vi "Configure.vi"(8 "error in":errorcluster, 10 "name":string="CRDS", 11 "tCRD in":refnum<class "tCRD.lvclass">) -> (0 "error out":errorcluster, 3 "tCRD out":refnum<class "tCRD.lvclass">)   [LabVIEW 2015, in "tCRD.lvclass"]
doc: "Configures the CRDS for operation and starts all DAQmx tasks associated with the instrument. This VI overrides the parent VI in the Instrument class."
uses:
  tCRD.lvclass
  Reusable/CRDS/Main/CRDS.lvclass
  Reusable/Instrument/Instrument.lvclass
  Reusable/Instrument/state.ctl
  Devices/Alicat/Session Based/Alicat Device.lvclass
  <userlib>/_Session Fwk/Session - Root.lvclass
  Reusable/Session APIs/File Access/Config Data/Config Session.ctl
  Reusable/Session APIs/File Access/Config Data/Config Data.lvclass
  Reusable/Session APIs/Serial/Serial Session.lvclass
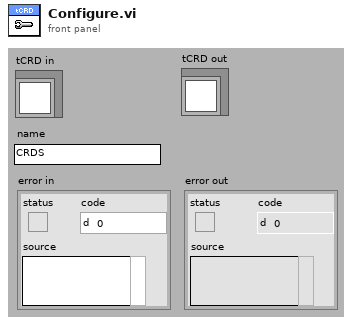
[diagram p1: front panel]
types:
  T1 = typedef "Config Data.lvclass/Config Session.ctl" = refnum<data-value>
  T2 = typedef "Instrument.lvclass/state.ctl" = enum8{"Configure", "Acquire", "Wait", "Quit", "Handle Error", "NOOP"}
  T3 = typedef "Session - Root.lvclass/Session Handle.ctl" = refnum<data-value>
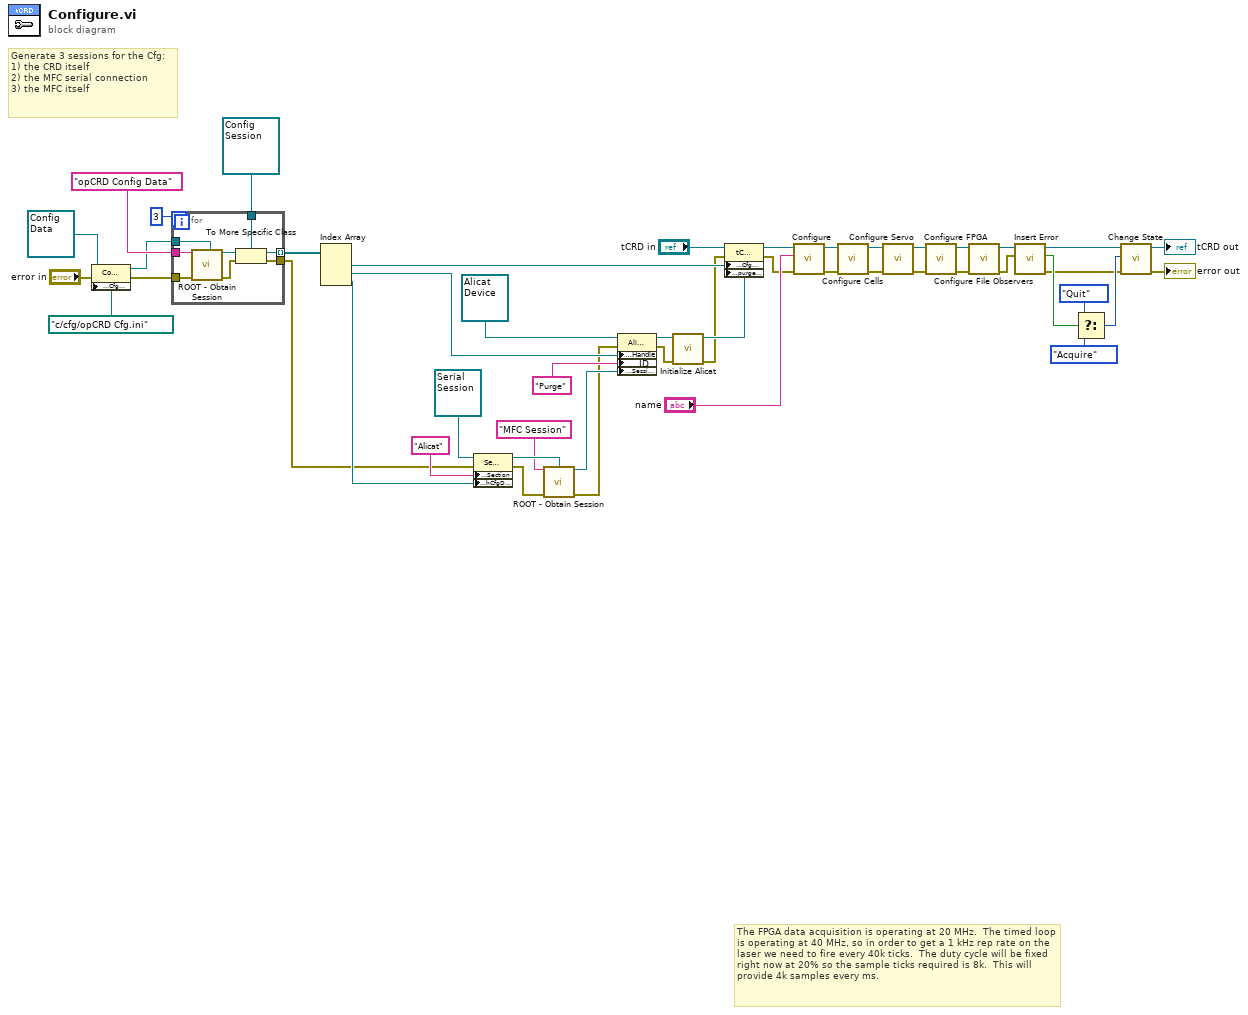
[diagram p0: block diagram]
diagram:
  # "Generate 3 sessions for the Cfg:\n1) the CRD itself\n2) the MFC serial connection\n3) the MFC itself"
  # "The FPGA data acquisition is operating at 20 MHz.  The timed loop is operating at 40 MHz, so in order to get a 1 kHz rep rate on the laser we need to fire every 40k ticks.  The duty cycle will be fixed right now at 20% so the sample ticks required is 8k.  This will provide 4k samples every ms."
  n1 = property class="Config Data"(reference=refnum<class "Config Data.lvclass"> refnum ("Config Data"), error in="error in", "Accessors:Cfg Path"=path "c:/cfg/opCRD Cfg.ini" ("Path")) -> (reference out=w18:refnum<class "Config Data.lvclass">, error out=w19:errorcluster)
  n2 = for {
    N: 3 -> [_]
    tunnel: [w55] -> w26 mode=indexing
    tunnel: "opCRD Config Data" ("Session Name ()") -> [w51]
    tunnel: T1 refnum ("Session Handle") -> [w50]
    tunnel: w19 -> [w53]
    tunnel: [w54] -> w4
    tunnel: w18 -> [w49]
    n3 = call <userlib>:"ROOT - Obtain Session.vi"("Session Name ()"=w51, "OBJ - Session"=w49, "error in (no error)"=w53) -> ("Session Handle"=w56:T3, "error out"=w52:errorcluster)  [unwired: 10 in, 1 out]
    n4 = To More Specific Class(target class=w50, reference=w56, error in=w52) -> (specific class reference=w55:T1, error out=w54:errorcluster)
  }
  n5 = Index Array(array=w26) -> (element #1=w7:T1, element #2=w16:T1, element #3=w15:T1)  [unwired: 3 in]
  n6 = property class="Serial Session"(reference=refnum<class "Serial Session.lvclass"> refnum ("Serial Session"), error in=w4, "Accessors:Section"="Alicat" ("Section"), "Accessors:hCfgData"=w15) -> (reference out=w31:refnum<class "Serial Session.lvclass">, error out=w28:errorcluster)
  n7 = call <userlib>:"ROOT - Obtain Session.vi"("Session Name ()"="MFC Session", "OBJ - Session"=w31, "error in (no error)"=w28) -> ("Session Handle"=w29:T3, "error out"=w3:errorcluster)  [unwired: 10 in, 1 out]
  n8 = property class="Alicat Device"(reference=refnum<class "Alicat Device.lvclass"> refnum ("Alicat Device in"), error in=w3, "Accessors:Handle"=w16, "Accessors:ID"="Purge", "Accessors:Session Handle"=w29) -> (reference out=w36:refnum<class "Alicat Device.lvclass">, error out=w35:errorcluster)
  n9 = call "Initialize Alicat.vi"("error in"=w35, "Alicat Device In"=w36) -> ("error out"=w2:errorcluster, "Alicat Device Out"=w6:refnum<class "Alicat Device.lvclass">)  [unwired: 8 in]
  n10 = property class="tCRD"(reference="tCRD in", error in=w2, "Accessors:Cfg Session"=w7, "Accessors:purgeFlow"=w6) -> (reference out=w8:refnum<class "tCRD.lvclass">, error out=w5:errorcluster)
  n11 = call-parent "Configure.vi"("error in"=w5, "name"="name", "CRDS in"=w8) -> ("error out"=w17:errorcluster, "CRDS out"=w10:refnum<class "tCRD.lvclass">)  [unwired: 7 in]
  n12 = call "Configure Cells.vi"("error in"=w17, "tCRD in"=w10) -> ("error out"=w1:errorcluster, "tCRD out"=w39:refnum<class "tCRD.lvclass">)  [unwired: 8 in]
  n13 = call "Configure Servo.vi"("error in"=w1, "tCRD in"=w39) -> ("error out"=w38:errorcluster, "tCRD out"=w40:refnum<class "tCRD.lvclass">)  [unwired: 8 in]
  n14 = call "Configure FPGA.vi"("error in"=w38, "tCRD in"=w40) -> ("error out"=w13:errorcluster, "tCRD out"=w14:refnum<class "tCRD.lvclass">)  [unwired: 8 in]
  n15 = call "Configure File Observers.vi"("error in"=w13, "tCRD in"=w14) -> ("error out"=w11:errorcluster, "tCRD out"=w12:refnum<class "tCRD.lvclass">)  [unwired: 8 in]
  n16 = call "Insert Error.vi"("err"=w11, "Instrument in"=w12) -> ("error out"=w42:errorcluster, "error?"=w45:bool, "Instrument out"=w43:refnum<class "tCRD.lvclass">)  [unwired: 7 in]
  n17 = Select(t=state."Quit" ("instr state"), s=w45, f=state."Acquire" ("instr state")) -> (s? t:f=w44:T2)
  n18 = call "Change State.vi"("error in"=w42, "instr state"=w44, "Instrument in"=w43) -> ("error out"=→"error out":errorcluster, "Instrument out"=→"tCRD out":refnum<class "tCRD.lvclass">)  [unwired: 7 in]
